vi "while_v0_v17.vi"() -> ()   [LabVIEW 2009]
panel:
  in  "Poz x":u16(slide)=136 scale=0.0..400.0
  in  "Poz y":u16(slide)=166 scale=300.0..0.0
  in  "Culoare":u32(colorbox)=16711713
  in  "Raza":u16(knob)=105 scale=0.0..200.0
  in  "stop":bool
  out "Picture":picture
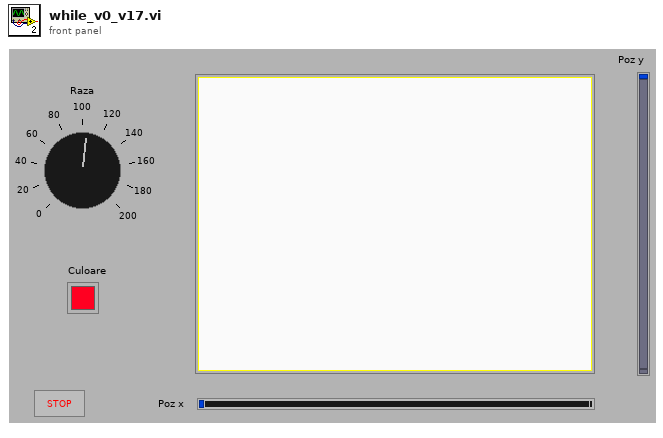
[diagram p1: front panel]
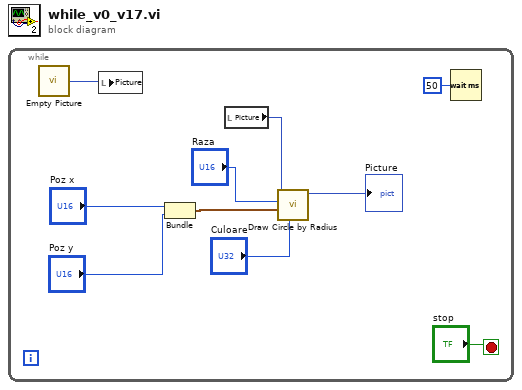
[diagram p0: block diagram]
diagram:
  n1 = while {
    stop <- "stop" stop-if-true
    n2 = call "Empty Picture"() -> ("empty picture"=w5:picture)
    n3 = local write "Picture"(w5) -> ()
    n4 = Bundle("Poz x"="Poz x", "Poz y"="Poz y") -> (w3:cluster{"Poz x":u16, "Poz y":u16})  [unwired: 1 in]
    n5 = local read "Picture"() -> (w9:picture)
    n6 = call <vilib>:"Draw Circle by Radius.vi"("color(black)"="Culoare", "pixel center"=w3, "radius"="Raza", "picture"=w9) -> ("new picture"=→"Picture":picture)  [unwired: 7 in]
    n7 = Wait (ms)(milliseconds to wait=u32 50) -> ()  [unwired: 1 out]
  }
